vi "Add Form.vi"(8 "error in (no error)":errorcluster, 9 "Nested":T1, 10 "Caller":T1, 11 "Autoclose manager in":refnum<class "Open Close Logic Simple Table.lvclass">) -> (0 "error out":errorcluster, 2 "Already opened?":bool, 3 "Autoclose manager out":refnum<class "Open Close Logic Simple Table.lvclass">)   [LabVIEW 2020, in "Open Close Logic Simple Table.lvlib" / "Open Close Logic Simple Table.lvclass"]
uses:
  Open Close Logic Simple Table.lvclass
  Form ID.ctl
  Open Close Logic Simple Table.lvclass/Open Close Logic Simple Table.ctl
  <userlib>/_OpenG.lib/array/array.llb/Search 1D Array (Variant)__ogtk.vi
  Form Server Interfaces.lvlib
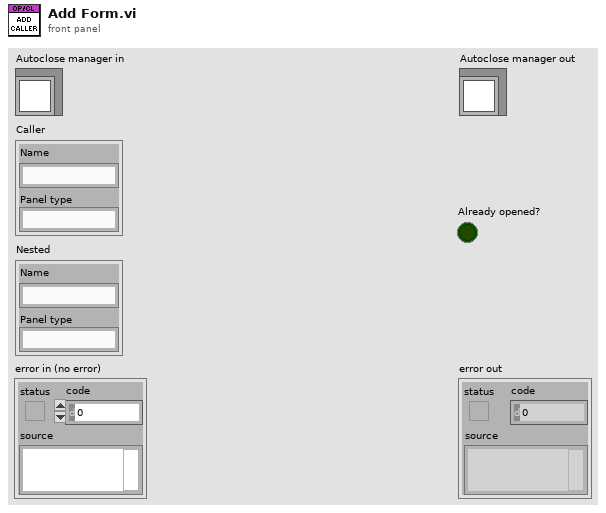
[diagram p1: front panel]
types:
  T1 = typedef "Form Server Interfaces.lvlib/Form ID.ctl" = cluster{"Name":string, "Panel type":string}
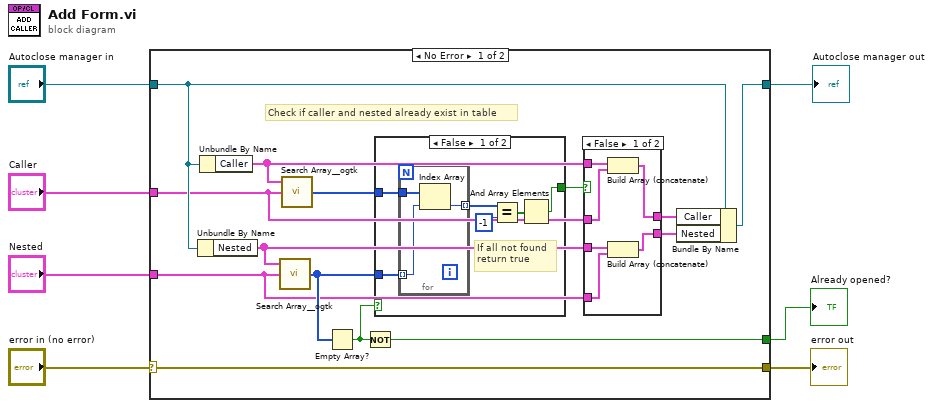
[diagram p0: block diagram]
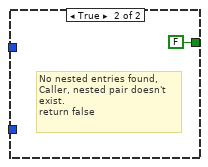
[diagram p3: hidden frame]
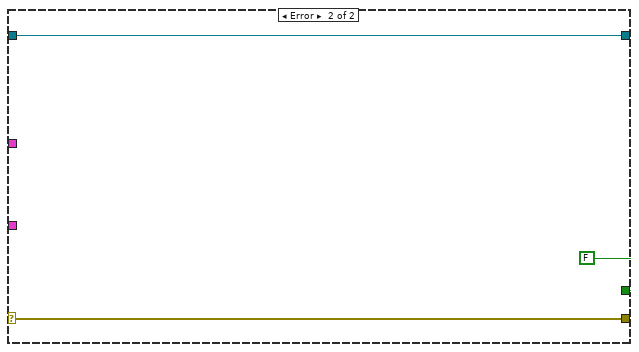
[diagram p4: hidden frame]
diagram:
  n1 = case shown="No Error" "error in (no error)" {
    selector: "error in (no error)" -> [w21 w41]
    tunnel: [w21 w41] -> w6
    tunnel: "Autoclose manager in" -> [w19 w42]
    tunnel: [w20 w42] -> w4
    tunnel: "Nested" -> [w10 _]
    tunnel: "Caller" -> [w11 _]
    tunnel: [w15 FALSE ("empty?")] -> w1
    frame No Error {
      # "Check if caller and nested already exist in table"
      n2 = Unbundle By Name(w19) -> ("Nested"=w12:T1[])
      n3 = Unbundle By Name(w19) -> ("Caller"=w13:T1[])
      n4 = call-poly <userlib>:"Search Array__ogtk.vi"("Array"=w12, "Element Data"=w10) -> ("Indices of Elements"=w18:i32[])  [unwired: 7 in]
      n5 = call-poly <userlib>:"Search Array__ogtk.vi"("Array"=w13, "Element Data"=w11) -> ("Indices of Elements"=w17:i32[])  [unwired: 7 in]
      n6 = Empty Array?(array=w18) -> (empty?=w16:bool)
      n7 = Not(x=w16) -> (.not. x?=w15:bool)
      n8 = case shown="False" w16 {
        tunnel: w18 -> [w35 _]
        tunnel: w17 -> [w34 _]
        tunnel: [w30 FALSE] -> w14
        frame False {
          # "If all not found\nreturn true"
          n9 = for {
            tunnel: w35 -> [w37] mode=indexing
            tunnel: w34 -> [w38]
            tunnel: [w36] -> w33 mode=indexing
            n10 = Index Array(array=w38, index=w37) -> (element=w36:i32)
          }
          n11 = Equal?(x=w33, y=-1) -> (x = y?=w31:bool[])
          n12 = And Array Elements(Boolean array=w31) -> (logical AND=w30:bool)
        }
        frame True {
          # "No nested entries found, Caller, nested pair doesn't exist.\nreturn false"
        }
      }
      n13 = case shown="False" w14 {
        tunnel: w13 -> [w27 w29]
        tunnel: w12 -> [w24 w28]
        tunnel: w11 -> [w26 _]
        tunnel: w10 -> [w23 _]
        tunnel: [w25 w29] -> w9
        tunnel: [w22 w28] -> w8
        frame False {
          n14 = Build Array (concatenate)(w27, w26) -> (w25:T1[])
          n15 = Build Array (concatenate)(w24, w23) -> (w22:T1[])
        }
        frame True {
        }
      }
      n16 = Bundle By Name(cluster=w19, "Caller"=w9, "Nested"=w8) -> (w20:refnum<class "Open Close Logic Simple Table.lvclass">)
    }
    frame Error {
    }
  }
  "error out" <- w6
  "Autoclose manager out" <- w4
  "Already opened?" <- w1
